vi "Demo Stop.vi"(8 "error in":errorcluster, 11 "UART port in":T1) -> (0 "error out":errorcluster, 3 "UART port out":T1)   [LabVIEW 2013]
doc: "Terminate the execution of a pre-configured demo.\n\nThis VI writes to, but does not read from, the serial port."
uses:
  UART/iRobot UART Port Type.ctl
  OpCode.ctl
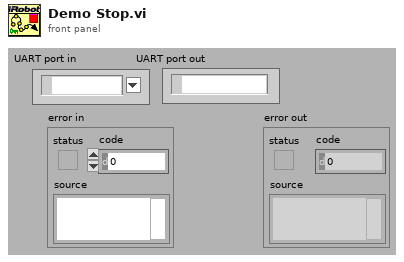
[diagram p1: front panel]
types:
  T1 = typedef "iRobot UART Port Type.ctl" = refnum<visa-resource-name>
  T2 = typedef "OpCode.ctl" = u8
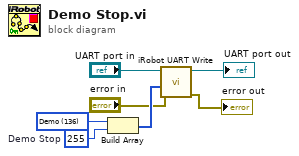
[diagram p0: block diagram]
diagram:
  w6 = u8 255  # Demo Stop
  w7 = T2 136 items=["Start"=128, "Baud"=129, "Control"=130, "Safe"=131, "Full"=132, "Demo"=136, "Demo - Cover"=135, "Demo - Cover and Dock"=143, "Demo - Spot"=134, "Drive"=137, "Drive Direct"=145, "LEDs"=139, "Digital Outputs"=147, "PWM Low Side Drivers"=144, "Low Side Drivers"=138, "Send IR"=151, "Song"=140, "Play Song"=141, "Sensors"=142, "Query List"=149, "Stream"=148, "Pause/Resume Stream"=150, "Script"=152, "Play Script"=153, "Show Script"=154, "Wait Time"=155, "Wait Distance"=156, "Wait Angle"=157, "Wait Event"=158] ("OpCode")
  n1 = Build Array(w7, w6) -> (w5:T2[])
  n2 = call "iRobot UART Write.vi"("error in"="error in", "data"=w5, "UART port in"="UART port in") -> ("error out"=→"error out":errorcluster, "UART port out"=→"UART port out":T1)  [unwired: 7 in]
